vi "RG lamp.vi"() -> ()   [LabVIEW 2018]
uses:
  lamp_state.ctl
panel:
  out "Rand Num":dbl
  in  "Exit":bool
  in  "Lamp init":bool
  in  "Generation Stop":bool
  in  "Generate Numbers":bool
  out "Green":bool
  out "Red":bool
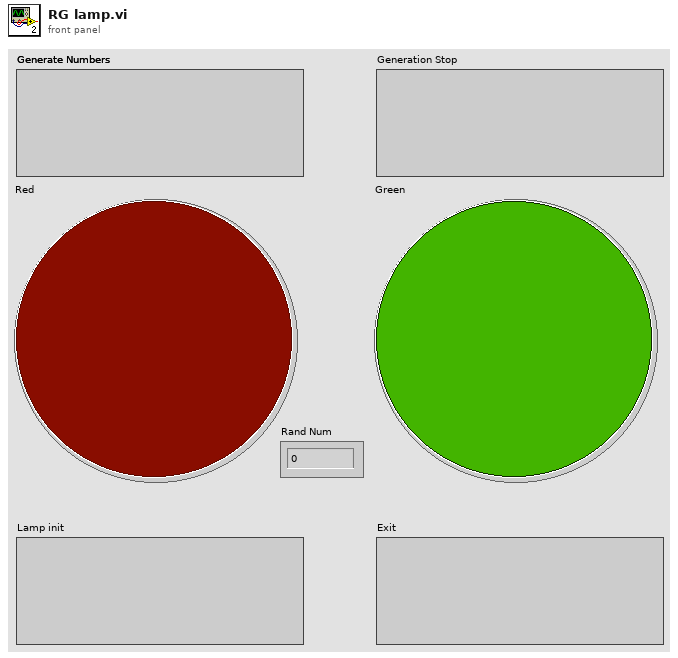
[diagram p1: front panel]
types:
  T1 = typedef "lamp_state.ctl" = enum16{"start", "Lamp initialization", "idle state", "green lamp on", "red lamp on", "rand_Num generatation", "Stop"}
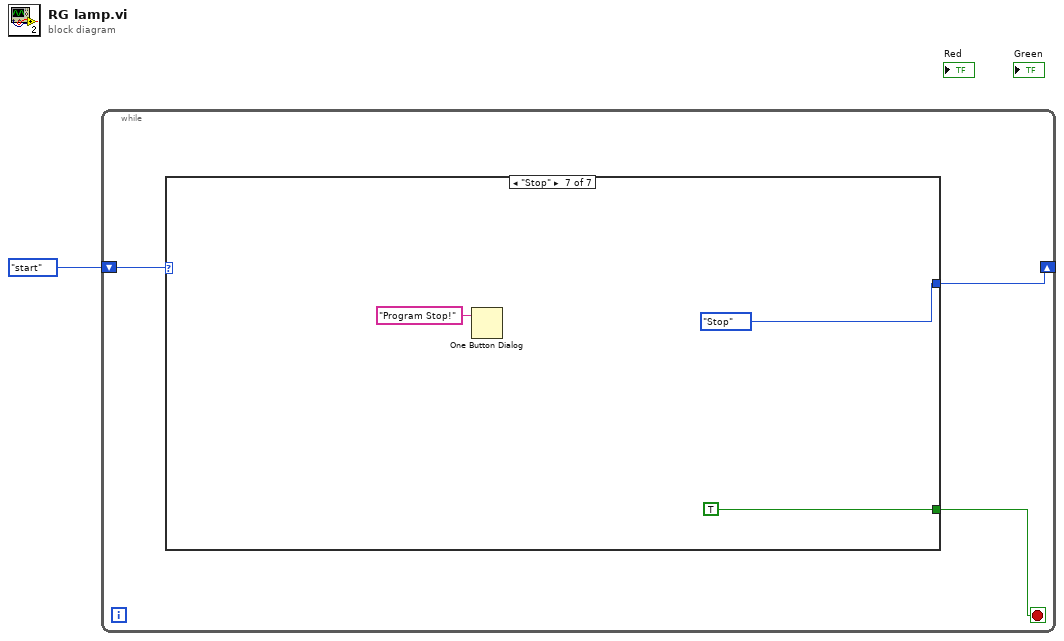
[diagram p0: block diagram]
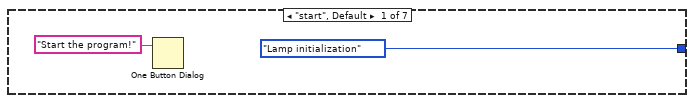
[diagram p2: hidden frame]
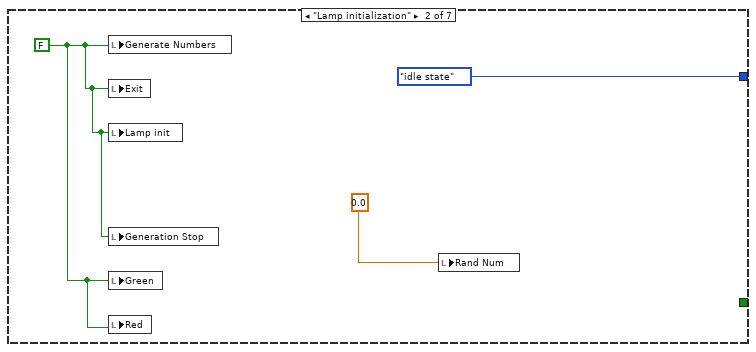
[diagram p3: hidden frame]
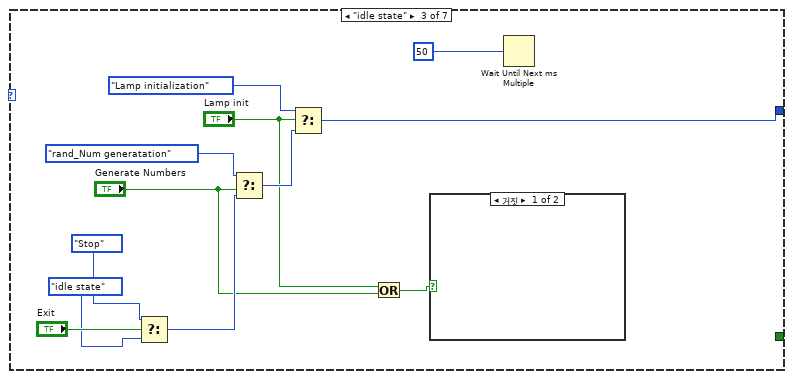
[diagram p4: hidden frame]
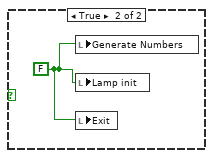
[diagram p5: hidden frame]
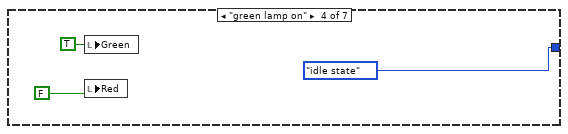
[diagram p6: hidden frame]
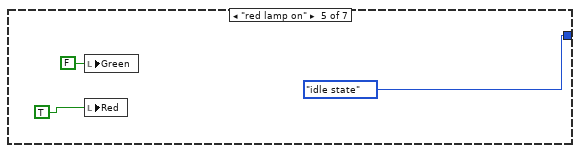
[diagram p7: hidden frame]
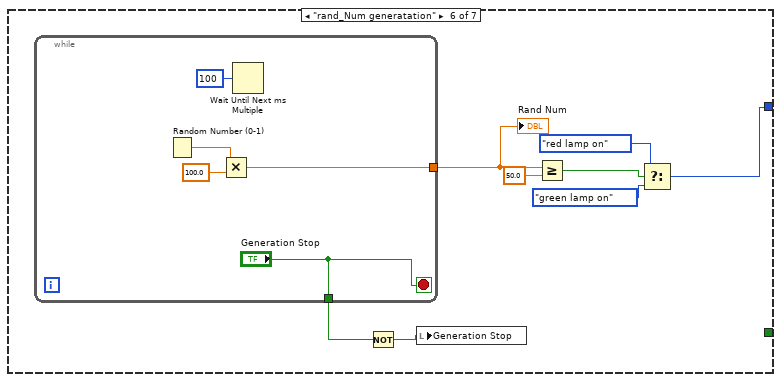
[diagram p8: hidden frame]
diagram:
  n1 = while {
    shift-right: [w3] -> _
    shift-left: lamp_state."start" ("열거형 2") -> [w4]
    stop <- w2 stop-if-true
    n2 = case shown="\"Stop\"" w4 {
      tunnel: [lamp_state."Lamp initialization" ("열거형 2") lamp_state."idle state" ("열거형 2") w14 lamp_state."idle state" ("열거형 2") lamp_state."idle state" ("열거형 2") w29 lamp_state."Stop" ("열거형 2")] -> w3
      tunnel: [_ _ _ _ _ _ TRUE] -> w2
      frame "start", Default {
        n3 = One Button Dialog(message="Start the program!" ("메시지")) -> ()  [unwired: 1 in, 1 out]
      }
      frame "Lamp initialization" {
        w9 = FALSE
        n4 = local write "Generate Numbers"(w9) -> ()
        n5 = local write "Exit"(w9) -> ()
        n6 = local write "Lamp init"(w9) -> ()
        n7 = local write "Generation Stop"(w9) -> ()
        n8 = local write "Green"(w9) -> ()
        n9 = local write "Red"(w9) -> ()
        n10 = local write "Rand Num"(0.0 ("Rand Num")) -> ()
      }
      frame "idle state" {
        n11 = Select(t=lamp_state."Stop" ("열거형 2"), s="Exit", f=lamp_state."idle state" ("열거형 2")) -> (s? t:f=w18:T1)
        n12 = Select(t=lamp_state."rand_Num generatation" ("열거형 2"), s="Generate Numbers", f=w18) -> (s? t:f=w16:T1)
        n13 = Select(t=lamp_state."Lamp initialization", s="Lamp init", f=w16) -> (s? t:f=w14:T1)
        n14 = Or(x="Lamp init", y="Generate Numbers") -> (x .or. y?=w11:bool)
        n15 = case shown="거짓" w11 {
          frame False {
          }
          frame True {
            w22 = FALSE
            n16 = local write "Generate Numbers"(w22) -> ()
            n17 = local write "Lamp init"(w22) -> ()
            n18 = local write "Exit"(w22) -> ()
          }
        }
        n19 = Wait Until Next ms Multiple(millisecond multiple=u32 50 ("ms 배수")) -> ()  [unwired: 1 out]
      }
      frame "green lamp on" {
        n20 = local write "Green"(TRUE ("Green")) -> ()
        n21 = local write "Red"(FALSE ("Green")) -> ()
      }
      frame "red lamp on" {
        n22 = local write "Green"(FALSE ("Green")) -> ()
        n23 = local write "Red"(TRUE ("Green")) -> ()
      }
      frame "rand_Num generatation" {
        n24 = while {
          tunnel: ["Generation Stop"] -> w36
          tunnel: [w37] -> w34
          stop <- "Generation Stop" stop-if-true
          n25 = Random Number (0-1)() -> (number: 0 to 1=w40:dbl)
          n26 = Multiply(x=w40, y=100.0) -> (x*y=w37:dbl)
          n27 = Wait Until Next ms Multiple(millisecond multiple=u32 100 ("ms 배수")) -> ()  [unwired: 1 out]
        }
        "Rand Num" <- w34
        n28 = Not(x=w36) -> (.not. x?=w35:bool)
        n29 = local write "Generation Stop"(w35) -> ()
        n30 = Greater Or Equal?(x=w34, y=50.0) -> (x >= y?=w32:bool)
        n31 = Select(t=lamp_state."red lamp on" ("열거형 2"), s=w32, f=lamp_state."green lamp on" ("열거형 2")) -> (s? t:f=w29:T1)
      }
      frame "Stop" {
        n32 = One Button Dialog(message="Program Stop!" ("메시지")) -> ()  [unwired: 1 in, 1 out]
      }
    }
  }
